vi "Inst_CNT90.vi"(8 "error in":errorcluster, 10 "All Message Queues in":T1, 11 "Prueba31 in":refnum<class "Prueba05.lvclass">) -> (0 "error out":errorcluster)   [LabVIEW 2019, in "Prueba05.lvclass"]
uses:
  Prueba05.lvclass
  QMH/Message Queue/All Message Queues.ctl
  QMH/Message Queue/Message Cluster.ctl
  Prueba05.lvclass/Prueba05.ctl
  <vilib>/Utility/error.llb/Error Cluster From Error Code.vi
  QMH/Message Queue/Enqueue Message (Single).vi
  <vilib>/ErrorRing/Error Ring.xnode
  QMH/Message Queue/Message Queue.lvlib
  Instrumento/CNT90/CNT90.lvclass
panel:
  out "All States":string[](array[string])
  out "Actual State":string
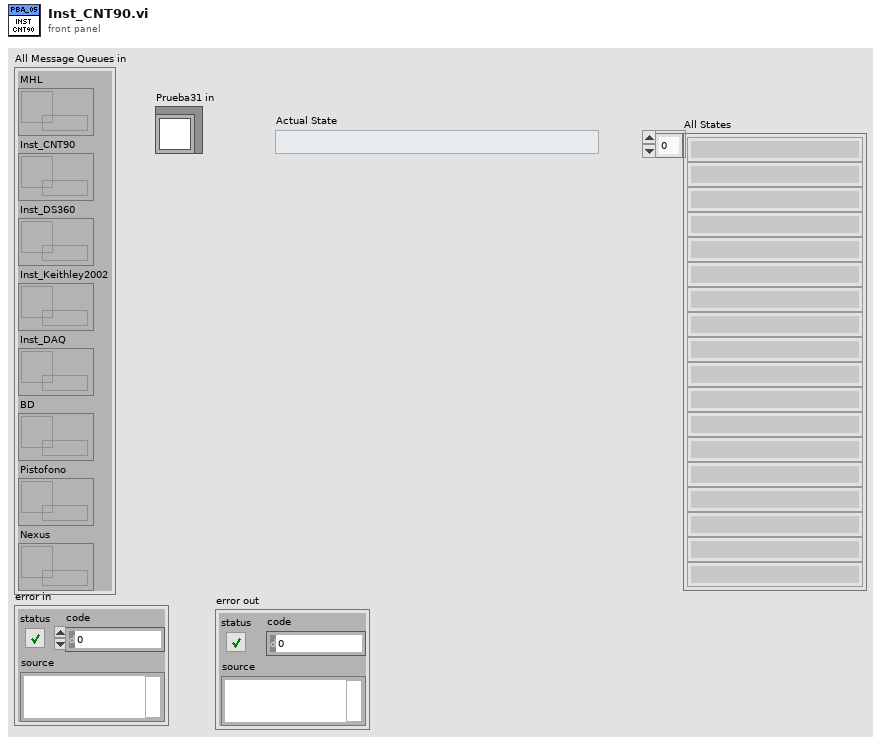
[diagram p1: front panel]
types:
  T1 = typedef "Message Queue.lvlib/All Message Queues.ctl" = cluster{"MHL":refnum<queue>, "Inst_CNT90":refnum<queue>, "Inst_DS360":refnum<queue>, "Inst_Keithley2002":refnum<queue>, "Inst_DAQ":refnum<queue>, "BD":refnum<queue>, "Pistofono":refnum<queue>, "Nexus":refnum<queue>}
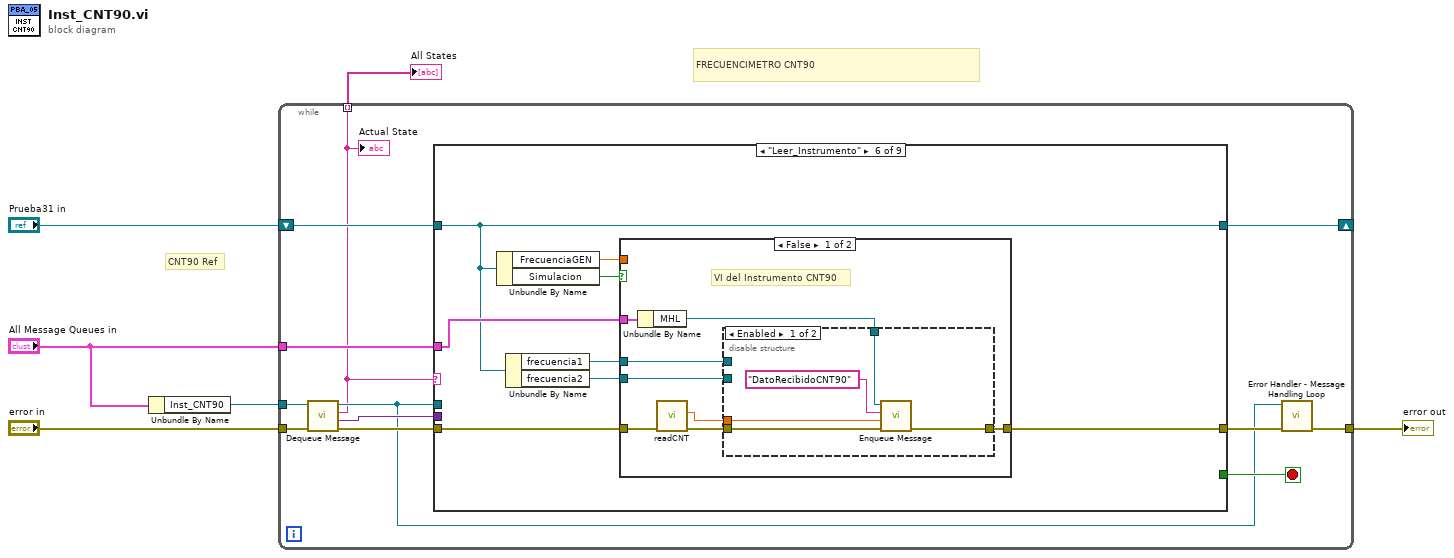
[diagram p0: block diagram]
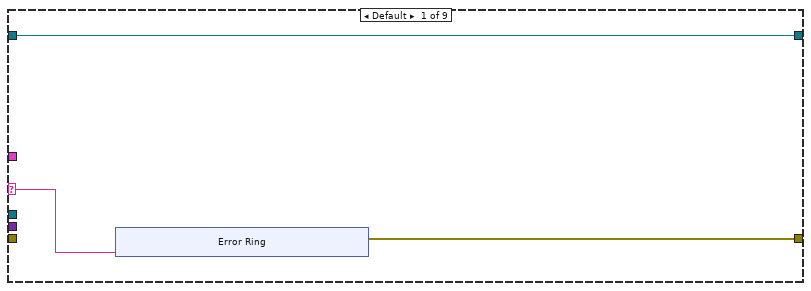
[diagram p2: hidden frame]
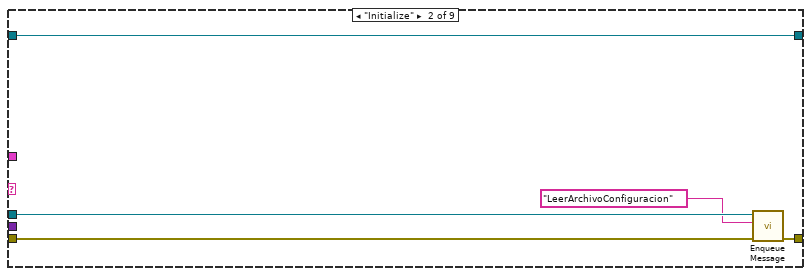
[diagram p3: hidden frame]
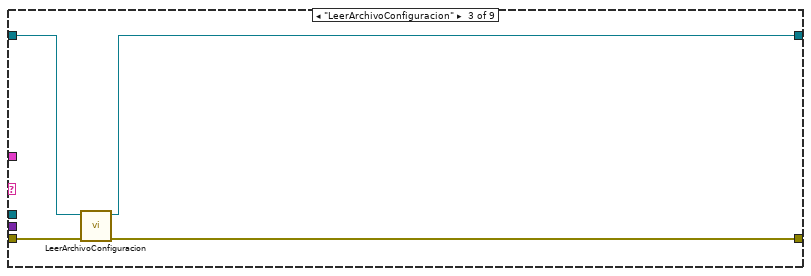
[diagram p4: hidden frame]
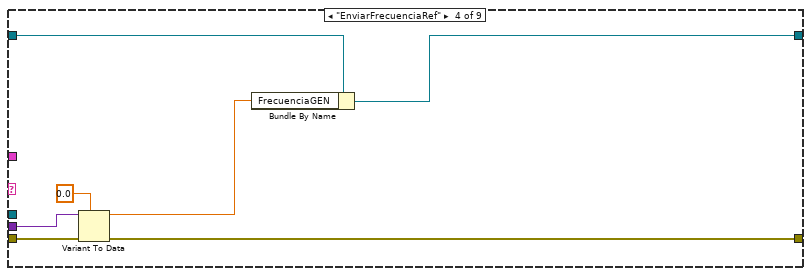
[diagram p5: hidden frame]
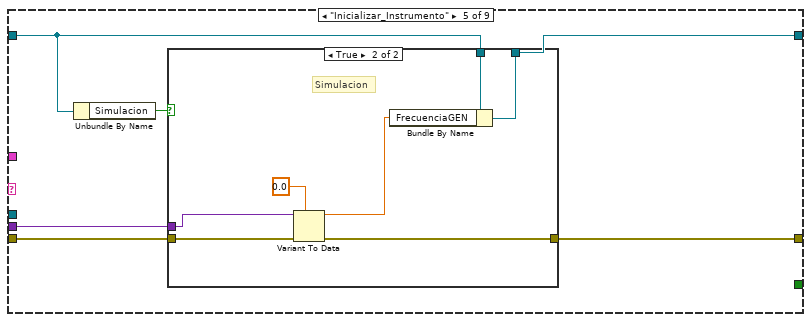
[diagram p6: hidden frame]
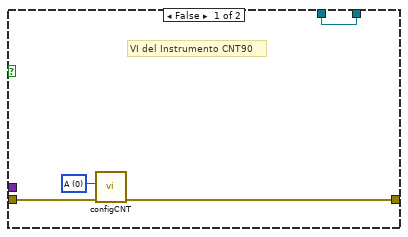
[diagram p7: hidden frame]
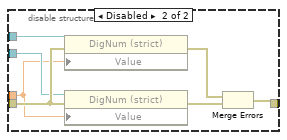
[diagram p8: hidden frame]
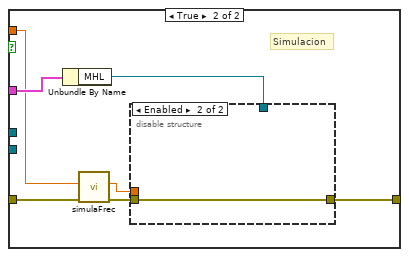
[diagram p9: hidden frame]
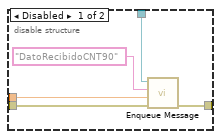
[diagram p10: hidden frame]
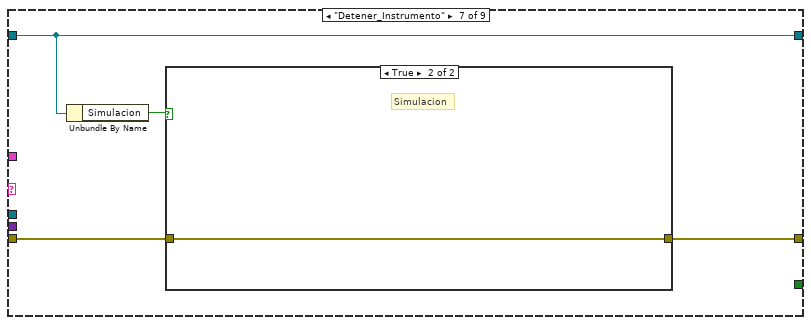
[diagram p11: hidden frame]
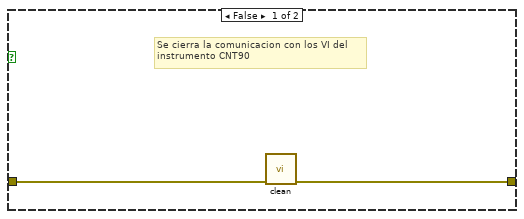
[diagram p12: hidden frame]
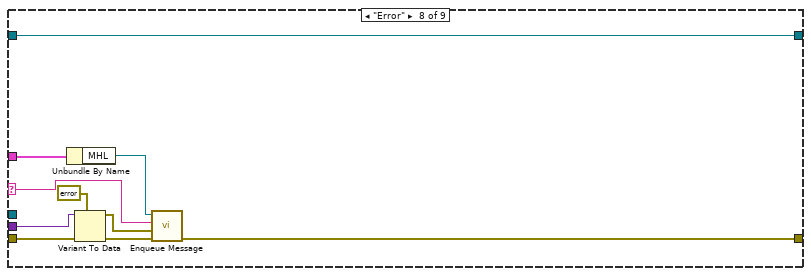
[diagram p13: hidden frame]
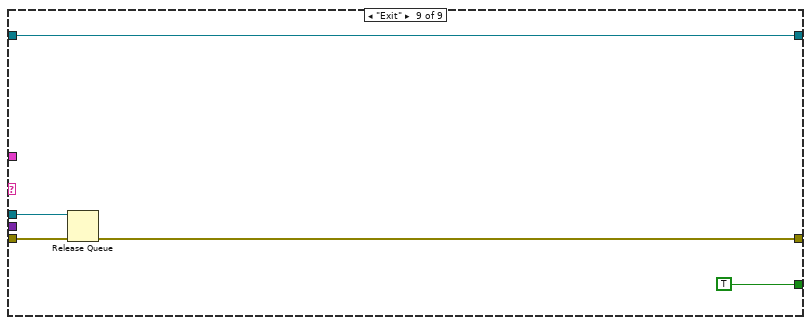
[diagram p14: hidden frame]
diagram:
  # "FRECUENCIMETRO CNT90"
  # "CNT90 Ref"
  n1 = Unbundle By Name("All Message Queues in") -> ("Inst_CNT90"=w4:refnum<queue>)
  n2 = while {
    tunnel: "error in" -> [w18]
    tunnel: w4 -> [w17]
    tunnel: "All Message Queues in" -> [w16]
    tunnel: [w9] -> w2
    shift-right: [w12] -> _
    shift-left: "Prueba31 in" -> [w15]
    tunnel: [w7] -> w1 mode=indexing
    stop <- w11 stop-if-true
    n3 = call "Dequeue Message.vi"("error in (no error)"=w18, "Message Queue"=w17) -> ("error out"=w13:errorcluster, "Message Data"=w14:variant, "Message"=w7:string, "dup Message Queue"=w8:refnum<queue>)  [unwired: 6 in]
    "Actual State" <- w7
    n4 = case shown="\"Leer_Instrumento\"" w7 {
      selector: w7 -> [w21 _ _ _ _ _ _ w114 _]
      tunnel: w16 -> [_ _ _ _ _ w66 _ w113 _]
      tunnel: w15 -> [w19 w33 w34 w39 w46 w64 w105 w111 w121]
      tunnel: w8 -> [_ w30 _ _ _ _ _ _ w123]
      tunnel: w14 -> [_ _ _ w42 w47 _ _ w117 _]
      tunnel: w13 -> [_ w31 w35 w43 w50 w69 w103 w118 w124]
      tunnel: [w20 w32 w37 w44 w48 w68 w106 w110 w120] -> w10
      tunnel: [w19 w33 w36 w40 w45 w64 w105 w111 w121] -> w12
      tunnel: [_ _ _ _ _ _ _ _ TRUE] -> w11
      frame Default {
        n5 = xnode "Error Ring"("parameter 0"=w21) -> ("error out"=w20:errorcluster)
      }
      frame "Initialize" {
        n6 = call-poly "Enqueue Message.vi"("error in (no error)"=w31, "Message"="LeerArchivoConfiguracion", "Message Queue"=w30) -> ("error out"=w32:errorcluster)  [unwired: 7 in, 1 out]
      }
      frame "LeerArchivoConfiguracion" {
        n7 = call "LeerArchivoConfiguracion.vi"("error in"=w35, "Prueba05 in"=w34) -> ("error out"=w37:errorcluster, "Prueba05 out"=w36:refnum<class "Prueba05.lvclass">)  [unwired: 8 in]
      }
      frame "EnviarFrecuenciaRef" {
        n8 = Variant To Data(error in=w43, type=0.0, Variant=w42) -> (data=w38:dbl, error out=w44:errorcluster)
        n9 = Bundle By Name(cluster=w39, "FrecuenciaGEN"=w38) -> (w40:refnum<class "Prueba05.lvclass">)
      }
      frame "Inicializar_Instrumento" {
        n10 = Unbundle By Name(w46) -> ("Simulacion"=w49:bool)
        n11 = case shown="True" w49 {
          tunnel: [w54 w60] -> w48
          tunnel: w50 -> [w53 w61]
          tunnel: w47 -> [_ w59]
          tunnel: w46 -> [w51 w57]
          tunnel: [w51 w56] -> w45
          frame False {
            w52 = 0 items=["A", "B"] ("Channel  1")
            # "VI del Instrumento CNT90"
            n12 = call "configCNT.vi"("error in (no error)"=w53, "Channel  1"=w52) -> ("error out"=w54:errorcluster)  [unwired: 8 in, 1 out]
          }
          frame True {
            # "Simulacion"
            n13 = Variant To Data(error in=w61, type=0.0, Variant=w59) -> (data=w55:dbl, error out=w60:errorcluster)
            n14 = Bundle By Name(cluster=w57, "FrecuenciaGEN"=w55) -> (w56:refnum<class "Prueba05.lvclass">)
          }
        }
      }
      frame "Leer_Instrumento" {
        n15 = Unbundle By Name(w64) -> ("FrecuenciaGEN"=w65:dbl, "Simulacion"=w67:bool)
        n16 = Unbundle By Name(w64) -> ("frecuencia1"=w63:refnum<vi>, "frecuencia2"=w62:refnum<vi>)
        n17 = case shown="False" w67 {
          tunnel: [w74 w96] -> w68
          tunnel: w69 -> [w77 w93]
          tunnel: w66 -> [w73 w95]
          tunnel: w65 -> [_ w90]
          tunnel: w63 -> [w71 _]
          tunnel: w62 -> [w70 _]
          frame False {
            # "VI del Instrumento CNT90"
            n18 = Unbundle By Name(w73) -> ("MHL"=w72:refnum<queue>)
            n19 = call "readCNT.vi"("error in (no error)"=w77) -> ("error out"=w75:errorcluster, "medicion"=w76:dbl)  [unwired: 8 in, 1 out]
            n20 = disable-structure shown="Enabled" {
              disable-tunnel: w76 -> [w82 w83]
              disable-tunnel: w75 -> [w80 w89]
              disable-tunnel: [w79 w88] -> w74
              disable-tunnel: w72 -> [w78 _]
              disable-tunnel: w71 -> [_ w85]
              disable-tunnel: w70 -> [_ w84]
              frame Enabled {
                n21 = call-poly "Enqueue Message.vi"("error in (no error)"=w80, "Message Data"=w82, "Message"="DatoRecibidoCNT90", "Message Queue"=w78) -> ("error out"=w79:errorcluster)  [unwired: 6 in, 1 out]
              }
              frame Disabled {
                n22 = property class="DigNum (strict)"(reference=w85, error in=w89, "Value"=w83) -> (error out=w86:errorcluster)  [unwired: 1 out]
                n23 = property class="DigNum (strict)"(reference=w84, error in=w89, "Value"=w83) -> (error out=w87:errorcluster)  [unwired: 1 out]
                n24 = Merge Errors(w86, w87) -> (w88:errorcluster)
              }
            }
          }
          frame True {
            # "Simulacion"
            n25 = Unbundle By Name(w95) -> ("MHL"=w94:refnum<queue>)
            n26 = call "simulaFrec.vi"("error in (no error)"=w93, "frec in"=w90) -> ("error out"=w92:errorcluster, "frec out"=w91:dbl)  [unwired: 7 in, 1 out]
            n27 = disable-structure shown="Enabled" {
              disable-tunnel: [w100 w102] -> w96
              disable-tunnel: w94 -> [w99 _]
              disable-tunnel: w92 -> [w98 w102]
              disable-tunnel: w91 -> [w97 _]
              frame Disabled {
                n28 = call-poly "Enqueue Message.vi"("error in (no error)"=w98, "Message Data"=w97, "Message"="DatoRecibidoCNT90", "Message Queue"=w99) -> ("error out"=w100:errorcluster)  [unwired: 6 in, 1 out]
              }
              frame Enabled {
              }
            }
          }
        }
      }
      frame "Detener_Instrumento" {
        n29 = Unbundle By Name(w105) -> ("Simulacion"=w104:bool)
        n30 = case shown="True" w104 {
          tunnel: [w108 w109] -> w106
          tunnel: w103 -> [w107 w109]
          frame False {
            # "Se cierra la comunicacion con los VI del\ninstrumento CNT90"
            n31 = call "clean.vi"("error in (no error)"=w107) -> ("error out"=w108:errorcluster)  [unwired: 9 in, 1 out]
          }
          frame True {
            # "Simulacion"
          }
        }
      }
      frame "Error" {
        n32 = Unbundle By Name(w113) -> ("MHL"=w112:refnum<queue>)
        n33 = Variant To Data(error in=w118, type=errorcluster {"status"=FALSE, "code"=0, "source"=""} ("error constant"), Variant=w117) -> (data=w115:errorcluster, error out=w116:errorcluster)
        n34 = call-poly "Enqueue Message.vi"("error in (no error)"=w116, "Message Data"=w115, "Message"=w114, "Message Queue"=w112) -> ("error out"=w110:errorcluster)  [unwired: 6 in, 1 out]
      }
      frame "Exit" {
        n35 = Release Queue(queue=w123, error in (no error)=w124) -> (error out=w120:errorcluster)  [unwired: 1 in, 2 out]
      }
    }
    n36 = call "Error Handler - Message Handling Loop.vi"("error in (no error)"=w10, "Message Queue"=w8) -> ("dup error in"=w9:errorcluster)  [unwired: 8 in, 1 out]
  }
  "error out" <- w2
  "All States" <- w1
